vi "Set Drive Output.vi"(6 "Rot. Point Y":dbl, 7 "Rot. Point X":dbl, 8 "Field Concentric":bool, 9 "Z":dbl(knob) scale=1.0..-1.0, 10 "Y":dbl(slide) scale=1.0..-1.0, 11 "X":dbl(slide) scale=-1.0..1.0) -> ()   [LabVIEW 2016]
uses:
  Robot Global Data.vi
panel:
  in  "Auto Controls":bool
  out "Number instances write":i32
  out "Number of Get":i32
  out "Array":dbl[](array[numeric])
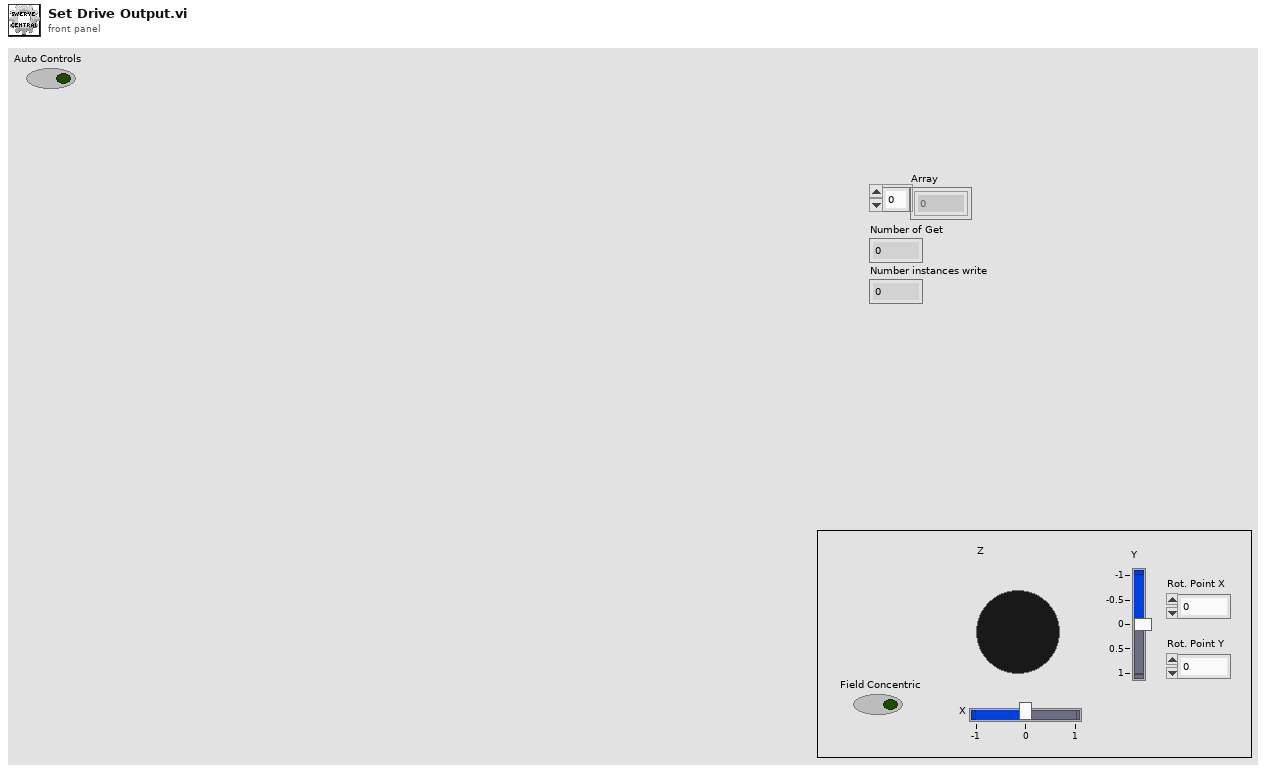
[diagram p1: front panel]
types:
  T1 = enum16{"FL Drive Wheel", "FR Drive Wheel", "RL Drive Wheel", "RR Drive Wheel", "FL Steer Wheel", "FR Steer Wheel", "RL Steer Wheel", "RR Steer Wheel"}
  T2 = typedef "WPI_MotorControlDeviceRef.ctl" = cluster{"DeviceStatus":errorcluster, "Type":T3, "PWM":cluster{"PWM Channel":T4, "DeadBand":T5}, "CAN":cluster{"Device Number":u8, "SetOutput VI Ref":variant, "GetOutput VI Ref":variant, "Enable VI Ref":variant, "Disable VI Ref":variant, "Data":variant}, "Invert":bool}
  T3 = typedef "WPI_MotorControlType.ctl" = enum16{"PWM", "CAN"}
  T4 = typedef "FPGA_DIOPWMChannel.ctl" = enum8{"PWM 0", "PWM 1", "PWM 2", "PWM 3", "PWM 4", "PWM 5", "PWM 6", "PWM 7", "PWM 8", "PWM 9", "PWM MXP 0", "PWM MXP 1", "PWM MXP 2", "PWM MXP 3", "PWM MXP 4", "PWM MXP 5", "PWM MXP 6", "PWM MXP 7", "PWM MXP 8", "PWM MXP 9", "Invalid"}
  T5 = typedef "WPI_PWMDeadband.ctl" = cluster{"Name":string, "maxPositivePwm":i32, "minPositivePwm":i32, "centerPwm":i32, "maxNegativePwm":i32, "minNegativePwm":i32, "angularRange":u16}
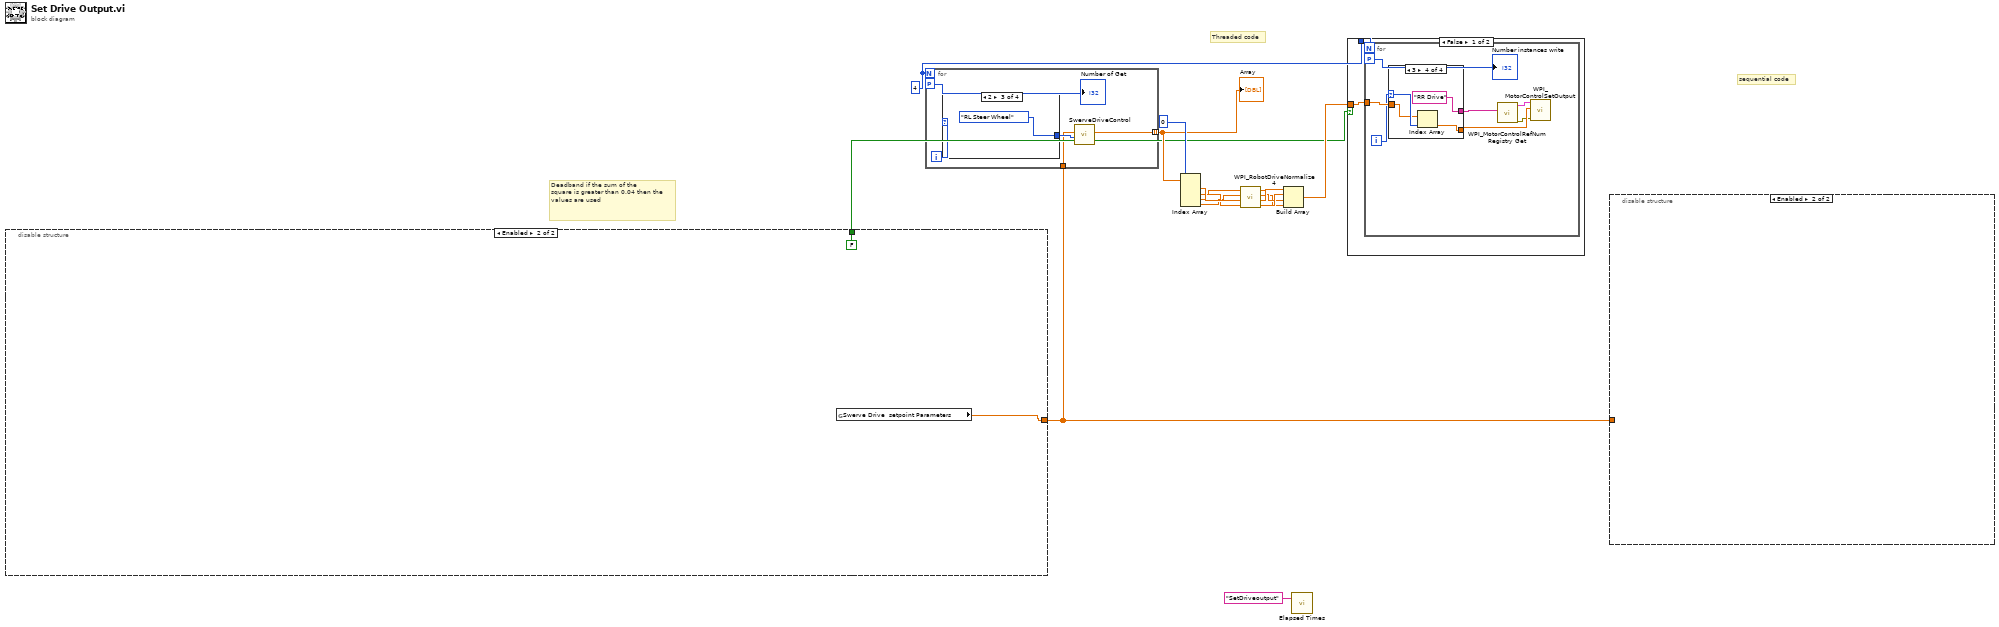
[diagram p0: block diagram]
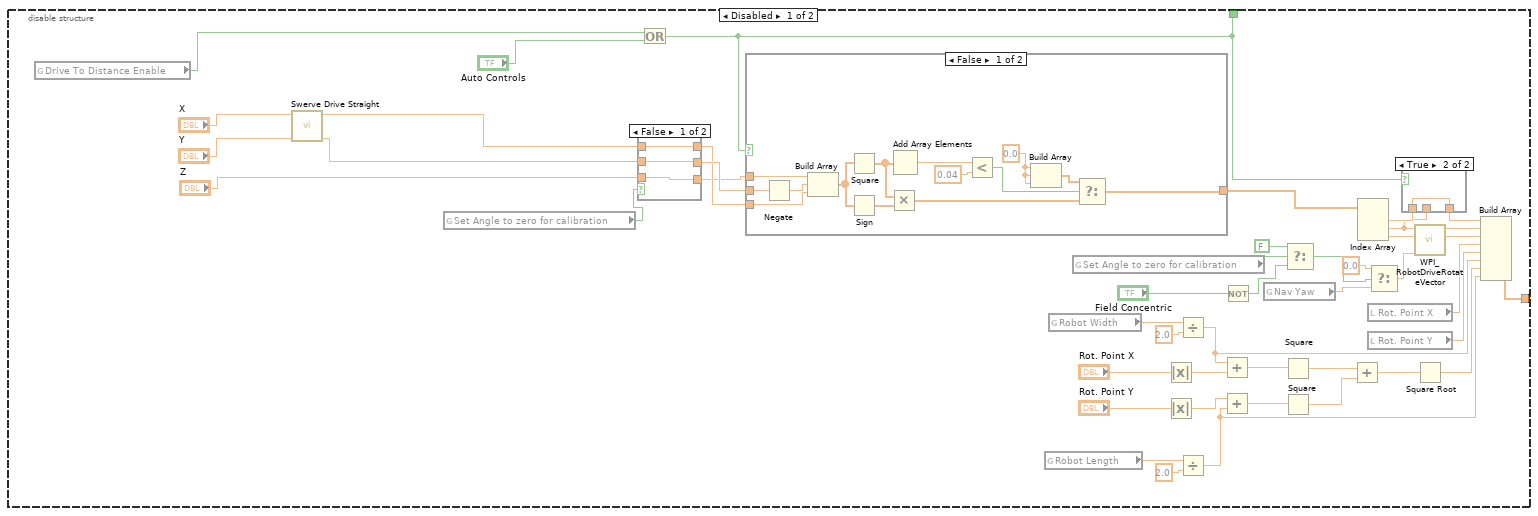
[diagram p2: hidden frame]
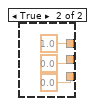
[diagram p3: hidden frame]
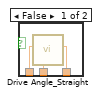
[diagram p4: hidden frame]
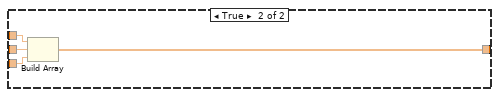
[diagram p5: hidden frame]
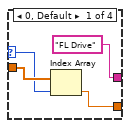
[diagram p6: hidden frame]
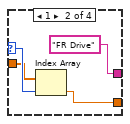
[diagram p7: hidden frame]
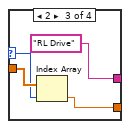
[diagram p8: hidden frame]
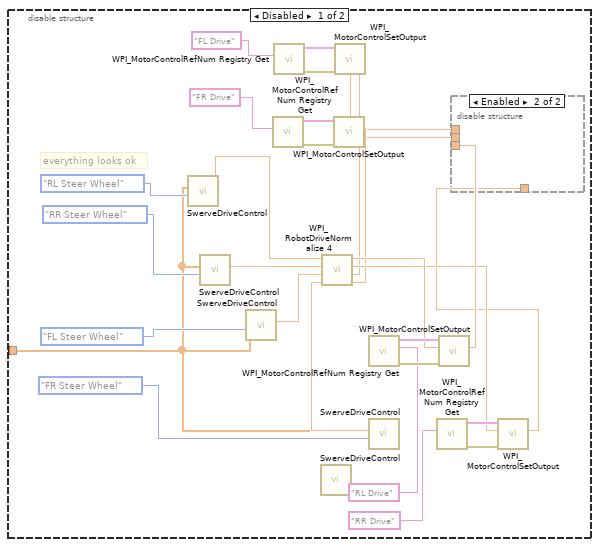
[diagram p10: hidden frame]
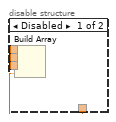
[diagram p11: hidden frame]
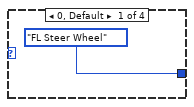
[diagram p12: hidden frame]
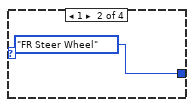
[diagram p13: hidden frame]
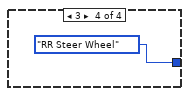
[diagram p14: hidden frame]
diagram:
  w2 = 4
  # "Threaded code"
  # "sequential code"
  # "Deadband if the sum of the \nsquare is greater than 0.04 then the \nvalues are used"
  n1 = disable-structure shown="Enabled" {
    disable-tunnel: [w36 w90] -> w14
    disable-tunnel: [w22 FALSE] -> w1
    frame Disabled {
      n2 = global read "Robot Global Data.vi" "Drive To Distance Enable"() -> (w20:bool)
      n3 = call "Swerve Drive Straight.vi"("Xin"="X", "Yin"="Y") -> ("Xout"=w16:dbl, "Yout"=w17:dbl)  [unwired: 7 in]
      n4 = global read "Robot Global Data.vi" "Set Angle to zero for calibration"() -> (w30:bool)
      n5 = case shown="False" w30 {
        tunnel: w17 -> [w64 _]
        tunnel: [w64 0.0 ("Y")] -> w33
        tunnel: w16 -> [w63 _]
        tunnel: [w63 1.0 ("X")] -> w32
        tunnel: "Z" -> [w62 _]
        tunnel: [w62 0.0 ("Z")] -> w31
        frame False {
        }
        frame True {
        }
      }
      n6 = Or(x=w20, y="Auto Controls") -> (x .or. y?=w22:bool)
      n7 = case shown="False" w22 {
        tunnel: [w75 w89] -> w61
        tunnel: w32 -> [w74 w88]
        tunnel: w31 -> [w72 w87]
        tunnel: w33 -> [w73 w86]
        frame False {
          w81 = 0.0 ("element")
          n8 = Negate(x=w73) -> (-x=w77:dbl)
          n9 = Build Array(w72, w77, w74) -> (w80:dbl[])
          n10 = Square(x=w80) -> (x^2=w78:dbl[])
          n11 = Sign(1:w80) -> (0:w79:dbl[])
          n12 = Multiply(x=w78, y=w79) -> (x*y=w76:dbl[])
          n13 = Add Array Elements(numeric array=w78) -> (sum=w85:dbl)
          n14 = Less?(x=w85, y=0.04 ("x")) -> (x < y?=w83:bool)
          n15 = Build Array(w81, w81, w81) -> (w82:dbl[])
          n16 = Select(t=w82, s=w83, f=w76) -> (s? t:f=w75:dbl[])
        }
        frame True {
          n17 = Build Array(w87, w86, w88) -> (w89:dbl[])
        }
      }
      n18 = global read "Robot Global Data.vi" "Robot Length"() -> (w39:dbl)
      n19 = global read "Robot Global Data.vi" "Robot Width"() -> (w40:dbl)
      n20 = global read "Robot Global Data.vi" "Set Angle to zero for calibration"() -> (w29:bool)
      n21 = Absolute Value(x="Rot. Point X") -> (abs(x)=w56:dbl)
      n22 = Absolute Value(x="Rot. Point Y") -> (abs(x)=w54:dbl)
      n23 = Divide(x=w40, y=2.0) -> (x/y=w45:dbl)
      n24 = Divide(x=w39, y=2.0) -> (x/y=w47:dbl)
      n25 = Add(x=w45, y=w56) -> (x+y=w55:dbl)
      n26 = Add(x=w54, y=w47) -> (x+y=w53:dbl)
      n27 = Not(x="Field Concentric") -> (.not. x?=w28:bool)
      n28 = global read "Robot Global Data.vi" "Nav Yaw"() -> (w58:dbl)
      n29 = Square(x=w55) -> (x^2=w51:dbl)
      n30 = Square(x=w53) -> (x^2=w52:dbl)
      n31 = Select(t=FALSE, s=w29, f=w28) -> (s? t:f=w27:bool)
      n32 = Add(x=w51, y=w52) -> (x+y=w50:dbl)
      n33 = Index Array(array=w61) -> (element #1=w35:dbl, element #2=w24:dbl, element #3=w25:dbl)  [unwired: 3 in]
      n34 = local read "Rot. Point X"() -> (w44:dbl)
      n35 = local read "Rot. Point Y"() -> (w43:dbl)
      n36 = Select(t=0.0, s=w27, f=w58) -> (s? t:f=w57:dbl)
      n37 = case shown="True" w22 {
        tunnel: w35 -> [w70 w71]
        tunnel: [w69 w71] -> w34
        tunnel: w24 -> [w68 _]
        frame False {
          n38 = call "Drive Angle_Straight.vi"("y input"=w68, "Z axis in"=w70) -> ("Z out"=w69:dbl)  [unwired: 9 in]
        }
        frame True {
        }
      }
      n39 = call <vilib>:"WPI_RobotDriveRotateVector.vi"("Angle"=w57, "X"=w25, "Y"=w24) -> ("X'"=w42:dbl, "Y'"=w41:dbl)  [unwired: 7 out]
      n40 = Square Root(x=w50) -> (sqrt(x)=w46:dbl)
      n41 = Build Array(w34, w41, w42, w44, w43, w45, w46, w47) -> (w36:dbl[])
    }
    frame Enabled {
      n42 = global read "Robot Global Data.vi" "Swerve Drive  setpoint Parameters"() -> (w90:dbl[])
    }
  }
  n43 = for {
    N: w2 -> [_]
    tunnel: [w93] -> w12 mode=indexing
    tunnel: w14 -> [w94]
    workers-P: _ -> [w92]
    i -> [w95]
    n44 = case shown="2" w95 {
      tunnel: [T1."FL Steer Wheel" ("Swerve Drive Param") T1."FR Steer Wheel" ("Swerve Drive Param") T1."RL Steer Wheel" ("Swerve Drive Param") T1."RR Steer Wheel" ("Swerve Drive Param")] -> w96
      frame 0, Default {
      }
      frame 1 {
      }
      frame 2 {
      }
      frame 3 {
      }
    }
    n45 = call "SwerveDriveControl.vi"("Swerve Drive Param"=w96, "Inputs"=w94) -> ("Speed"=w93:dbl)  [unwired: 9 in]
    "Number of Get" <- w92
  }
  "Array" <- w12
  n46 = Index Array(array=w12, index #1=0 ("index")) -> (element #1=w11:dbl, element #2=w10:dbl, element #3=w9:dbl, element #4=w8:dbl)  [unwired: 3 in]
  n47 = call <vilib>:"WPI_RobotDriveNormalize 4.vi"("D"=w10, "C"=w11, "B"=w8, "A"=w9) -> ("D'"=w6:dbl, "C'"=w7:dbl, "B'"=w4:dbl, "A'"=w5:dbl)
  n48 = Build Array(w7, w6, w5, w4) -> (w3:dbl[])
  n49 = call "Elapsed Times.vi"("Call Name"="SetDriveoutput") -> ()  [unwired: 2 in, 1 out]
  n50 = case shown="False" w1 {
    tunnel: w3 -> [w102 _]
    tunnel: w2 -> [w101 _]
    frame False {
      n51 = for {
        N: w101 -> [_]
        tunnel: w102 -> [w109]
        workers-P: _ -> [w105]
        i -> [w108]
        n52 = case shown="3" w108 {
          selector: w108 -> [w112 w117 w120 w125]
          tunnel: w109 -> [w113 w116 w121 w124]
          tunnel: ["FL Drive" ("refnum name") "FR Drive" ("refnum name") "RL Drive" ("refnum name") "RR Drive" ("refnum name")] -> w107
          tunnel: [w111 w115 w119 w122] -> w106
          frame 0, Default {
            n53 = Index Array(array=w113, index=w112) -> (element=w111:dbl)
          }
          frame 1 {
            n54 = Index Array(array=w116, index=w117) -> (element=w115:dbl)
          }
          frame 2 {
            n55 = Index Array(array=w121, index=w120) -> (element=w119:dbl)
          }
          frame 3 {
            n56 = Index Array(array=w124, index=w125) -> (element=w122:dbl)
          }
        }
        n57 = call <vilib>:"WPI_MotorControlRefNum Registry Get.vi"("refnum name"=w107) -> ("error out"=w103:errorcluster, "MotorControlDevRef"=w104:T2)  [unwired: 9 in]
        n58 = call <vilib>:"WPI_MotorControlSetOutput.vi"("error in (no error)"=w103, "Output"=w106, "MotorControlDevRef"=w104) -> ()  [unwired: 6 in, 3 out]
        "Number instances write" <- w105
      }
    }
    frame True {
    }
  }
  n59 = disable-structure shown="Enabled" {
    disable-tunnel: w14 -> [w126 _]
    frame Disabled {
      # "everything looks ok"
      n60 = call "SwerveDriveControl.vi"("Swerve Drive Param"=T1."RL Steer Wheel", "Inputs"=w126) -> ("Speed"=w138:dbl)  [unwired: 9 in]
      n61 = call "SwerveDriveControl.vi"("Swerve Drive Param"=T1."RR Steer Wheel", "Inputs"=w126) -> ("Speed"=w137:dbl)  [unwired: 9 in]
      n62 = call "SwerveDriveControl.vi"("Swerve Drive Param"=T1."FL Steer Wheel", "Inputs"=w126) -> ("Speed"=w136:dbl)  [unwired: 9 in]
      n63 = call <vilib>:"WPI_MotorControlRefNum Registry Get.vi"("refnum name"="FR Drive") -> ("error out"=w144:errorcluster, "MotorControlDevRef"=w142:T2)  [unwired: 9 in]
      n64 = call <vilib>:"WPI_MotorControlRefNum Registry Get.vi"("refnum name"="FL Drive") -> ("error out"=w146:errorcluster, "MotorControlDevRef"=w145:T2)  [unwired: 9 in]
      n65 = call "SwerveDriveControl.vi"() -> ()  [unwired: 11 in, 1 out]
      n66 = call <vilib>:"WPI_MotorControlRefNum Registry Get.vi"("refnum name"="RL Drive") -> ("error out"=w150:errorcluster, "MotorControlDevRef"=w149:T2)  [unwired: 9 in]
      n67 = call "SwerveDriveControl.vi"("Swerve Drive Param"=T1."FR Steer Wheel", "Inputs"=w126) -> ("Speed"=w135:dbl)  [unwired: 9 in]
      n68 = call <vilib>:"WPI_RobotDriveNormalize 4.vi"("D"=w135, "C"=w136, "B"=w137, "A"=w138) -> ("D'"=w131:dbl, "C'"=w132:dbl, "B'"=w133:dbl, "A'"=w134:dbl)
      n69 = call <vilib>:"WPI_MotorControlSetOutput.vi"("error in (no error)"=w144, "Output"=w131, "MotorControlDevRef"=w142) -> ("Motor Output"=w129:dbl)  [unwired: 6 in, 2 out]
      n70 = call <vilib>:"WPI_MotorControlSetOutput.vi"("error in (no error)"=w146, "Output"=w132, "MotorControlDevRef"=w145) -> ("Motor Output"=w130:dbl)  [unwired: 6 in, 2 out]
      n71 = call <vilib>:"WPI_MotorControlRefNum Registry Get.vi"("refnum name"="RR Drive") -> ("error out"=w148:errorcluster, "MotorControlDevRef"=w147:T2)  [unwired: 9 in]
      n72 = call <vilib>:"WPI_MotorControlSetOutput.vi"("error in (no error)"=w150, "Output"=w134, "MotorControlDevRef"=w149) -> ("Motor Output"=w128:dbl)  [unwired: 6 in, 2 out]
      n73 = call <vilib>:"WPI_MotorControlSetOutput.vi"("error in (no error)"=w148, "Output"=w133, "MotorControlDevRef"=w147) -> ("Motor Output"=w127:dbl)  [unwired: 6 in, 2 out]
      n74 = disable-structure shown="Enabled" {
        disable-tunnel: w130 -> [w158 _]
        disable-tunnel: w129 -> [w157 _]
        disable-tunnel: w128 -> [w156 _]
        disable-tunnel: w127 -> [w155 _]
        frame Disabled {
          n75 = Build Array(w158, w157, w156, w155) -> (w159:dbl[])
        }
        frame Enabled {
        }
      }
    }
    frame Enabled {
    }
  }
